vi "Get Signal Direction.vi"(8 "error in (no error)":errorcluster, 11 "IO Class in":refnum<class "IO Class.lvclass">) -> (0 "error out":errorcluster, 2 "Direction":enum16{"Input", "Output"}(ring), 3 "IO Class out":refnum<class "IO Class.lvclass">)   [LabVIEW 2015, in "IO Class.lvclass"]
uses:
  IO Class.lvclass
  Configuration.ctl
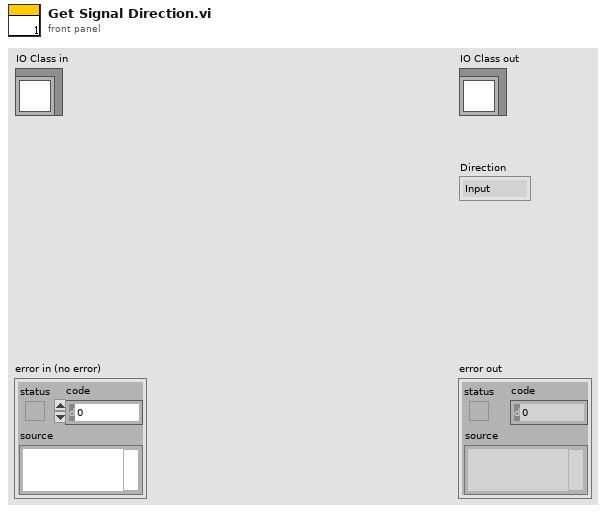
[diagram p1: front panel]
types:
  T1 = typedef "IO Class.lvclass/Configuration.ctl" = cluster{"Classification":string, "Direction":string, "Type":string}
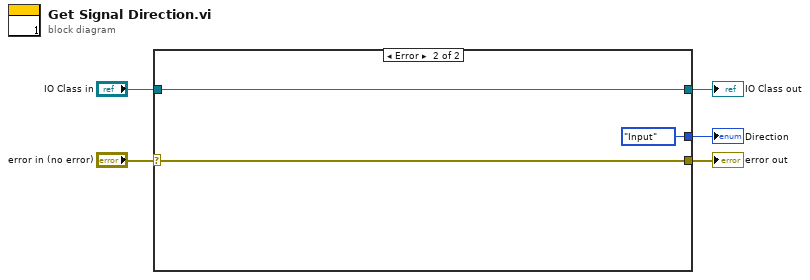
[diagram p0: block diagram]
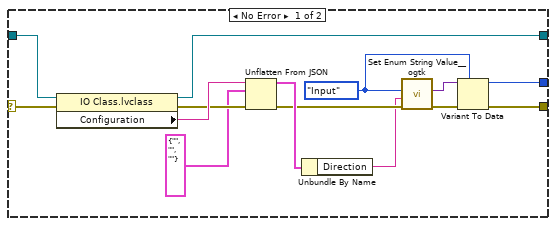
[diagram p2: hidden frame]
diagram:
  n1 = case shown="Error" "error in (no error)" {
    selector: "error in (no error)" -> [w10 w22]
    tunnel: [w9 w22] -> w4
    tunnel: [w6 w21] -> w2
    tunnel: "IO Class in" -> [w7 w21]
    tunnel: [w8 enum16{"Input", "Output"}."Input" ("Direction")] -> w1
    frame No Error {
      w12 = enum16{"Input", "Output"}."Input" ("Direction")
      n2 = property class="IO Class.lvclass"(reference=w7, error in=w10) -> (reference out=w6:refnum<class "IO Class.lvclass">, error out=w18:errorcluster, "Configuration"=w19:string)
      n3 = Unflatten From JSON(JSON string=w19, type and defaults=T1 {"Classification"="", "Direction"="", "Type"=""} ("Configuration"), error in (no error)=w18) -> (value=w17:T1, error out=w16:errorcluster)  [unwired: 4 in]
      n4 = Unbundle By Name(w17) -> ("Direction"=w15:string)
      n5 = call <userlib>:"Set Enum String Value__ogtk.vi"("error in (no error)"=w16, "String Value"=w15, "Default Enum Value"=w12) -> ("error out"=w14:errorcluster, "Enum"=w13:variant)  [unwired: 7 in]
      n6 = Variant To Data(error in=w14, type=w12, Variant=w13) -> (data=w8:enum16{"Input", "Output"}, error out=w9:errorcluster)
    }
    frame Error {
    }
  }
  "error out" <- w4
  "IO Class out" <- w2
  "Direction" <- w1
